vi "filter_01.vi"(2 "Раз":i32=1, 3 "SignalIn":waveform(i16)) -> (0 "error":i32, 1 "SignalOut":waveform(i16))   [LabVIEW 2010]
uses:
  <vilib>/Analysis/3filter.llb/Equi-Ripple BandStop (DBL).vi
  <vilib>/Analysis/NI_AALBase.lvlib
panel:
  in  "Что отобразить":u16(ring) items=["Вход", "Выход", "Оба"]
  in  "# of taps":i32=500
  out "Частота":dbl
  in  "Hp":dbl=500000.0
  in  "Hs":dbl=400000.0
  in  "Ls":dbl=200000.0
  in  "Lp":dbl=150000.0
  out "Осциллограмма 2":waveform(i16)[](graph)
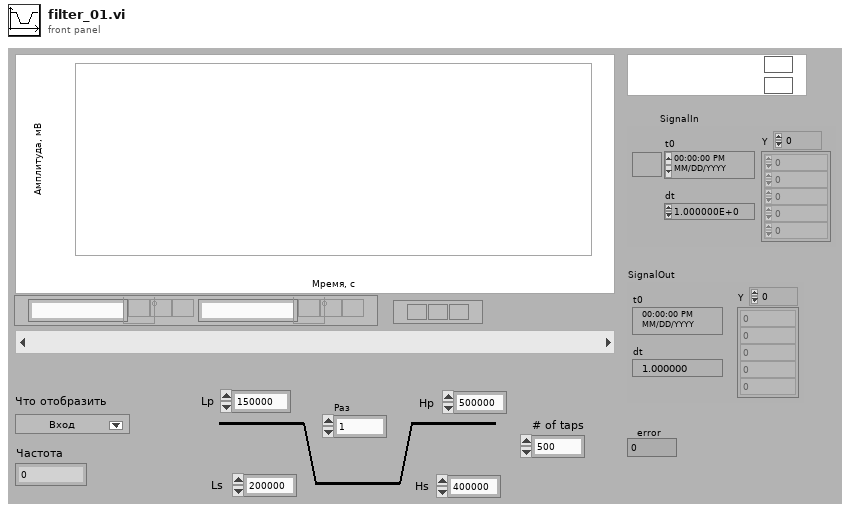
[diagram p1: front panel]
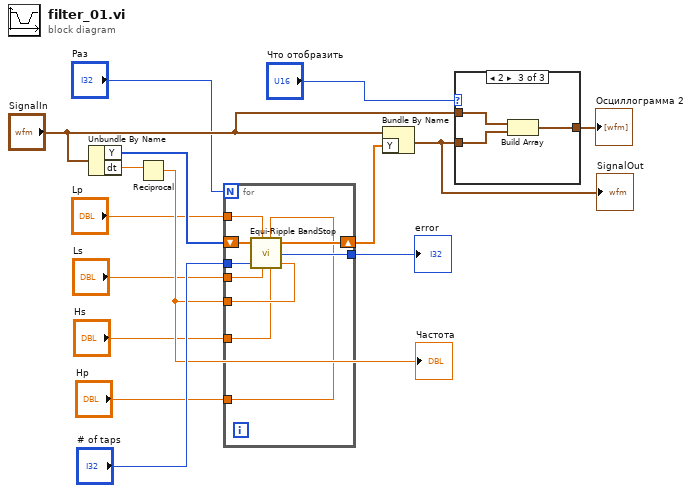
[diagram p0: block diagram]
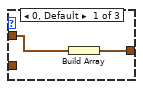
[diagram p2: hidden frame]
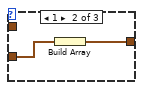
[diagram p3: hidden frame]
diagram:
  n1 = Unbundle By Name("SignalIn") -> ("Y"=w10:i16[], "dt"=w14:dbl)
  n2 = Reciprocal(x=w14) -> (1/x=w8:dbl)
  "Частота" <- w8
  n3 = for {
    N: "Раз" -> [_]
    tunnel: "# of taps" -> [w22]
    tunnel: w8 -> [w21]
    tunnel: [w20] -> w7
    tunnel: "Ls" -> [w19]
    tunnel: "Hs" -> [w18]
    tunnel: "Lp" -> [w17]
    tunnel: "Hp" -> [w16]
    shift-right: [w24] -> w11
    shift-left: w10 -> [w23]
    n4 = call-poly <vilib>:"Equi-Ripple BandStop.vi"("X"=w23, "lower pass freq"=w17, "# of taps"=w22, "lower stop freq"=w19, "higher pass freq"=w16, "higher stop freq"=w18, "sampling freq: fs"=w21) -> ("Filtered X"=w24:dbl[], "error"=w20:i32)  [unwired: 1 in]
  }
  "error" <- w7
  n5 = Bundle By Name(cluster="SignalIn", "Y"=w11) -> (w2:waveform(i16))
  "SignalOut" <- w2
  n6 = case shown="2" "Что отобразить" {
    tunnel: "SignalIn" -> [w26 _ w30]
    tunnel: w2 -> [_ w27 w29]
    tunnel: [w25 w28 w31] -> w12
    frame 0, Default {
      n7 = Build Array(w26) -> (w25:waveform(i16)[])
    }
    frame 1 {
      n8 = Build Array(w27) -> (w28:waveform(i16)[])
    }
    frame 2 {
      n9 = Build Array(w30, w29) -> (w31:waveform(i16)[])
    }
  }
  "Осциллограмма 2" <- w12
